vi "CSM - Destroy Broadcast Event.vi"(8 "Error In":errorcluster caption="error in (no error)", 11 "Broadcast Event":T1) -> (0 "error out":errorcluster)   [LabVIEW 2017, in "Communicable State Machine.lvlib"]
doc: "### CSM - Destroy Status Change Event.vi\n\nRelease the CSM status change event handle.\n\n-- <b>Controls</b> --\n- <b>Status Change Event</b>: CSM status change event handle"
uses:
  Communicable State Machine.lvlib
  _Support/Typedef/_CSM Status Change Event Data.ctl
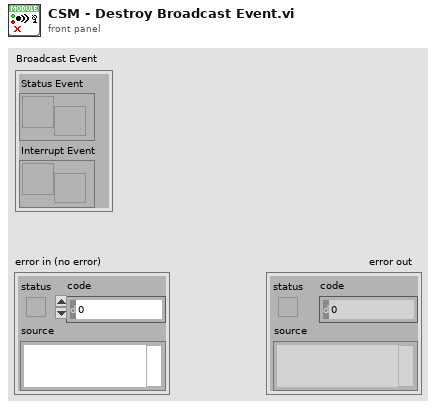
[diagram p1: front panel]
types:
  T1 = cluster{"Status Event":refnum<user-event>, "Interrupt Event":refnum<user-event>}
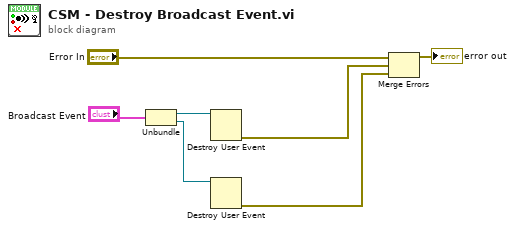
[diagram p0: block diagram]
diagram:
  n1 = Unbundle("Broadcast Event") -> ("Status Event"=w3:refnum<user-event>, "Interrupt Event"=w2:refnum<user-event>)
  n2 = Destroy User Event(user event=w3) -> (error out=w7:errorcluster)  [unwired: 1 in]
  n3 = Destroy User Event(user event=w2) -> (error out=w1:errorcluster)  [unwired: 1 in]
  n4 = Merge Errors("Error In", w7, w1) -> (→"error out":errorcluster)
